vi "Prueba.vi"() -> ()   [LabVIEW 2026]
uses:
  <vilib>/picture/picture.llb/imagedata.ctl
panel:
  out "return code":i32
  out "match + rest of string":string
  out "new picture":picture
  out "standard output":string
  in  "UPLOAD":bool
  in  "DOWNLOAD":bool
  in  "VER IMAGEN":bool
  in  "LEER ARCHIVO":bool
  in  "Single Selection Listbox":i32(listbox)
  out "Lista de archivos":string[](array[string])
  out "Enum":enum16{"ESPERAR", "LIST"}(ring)
  in  "stop":bool
  in  "LISTAR":bool
  in  "IP":string
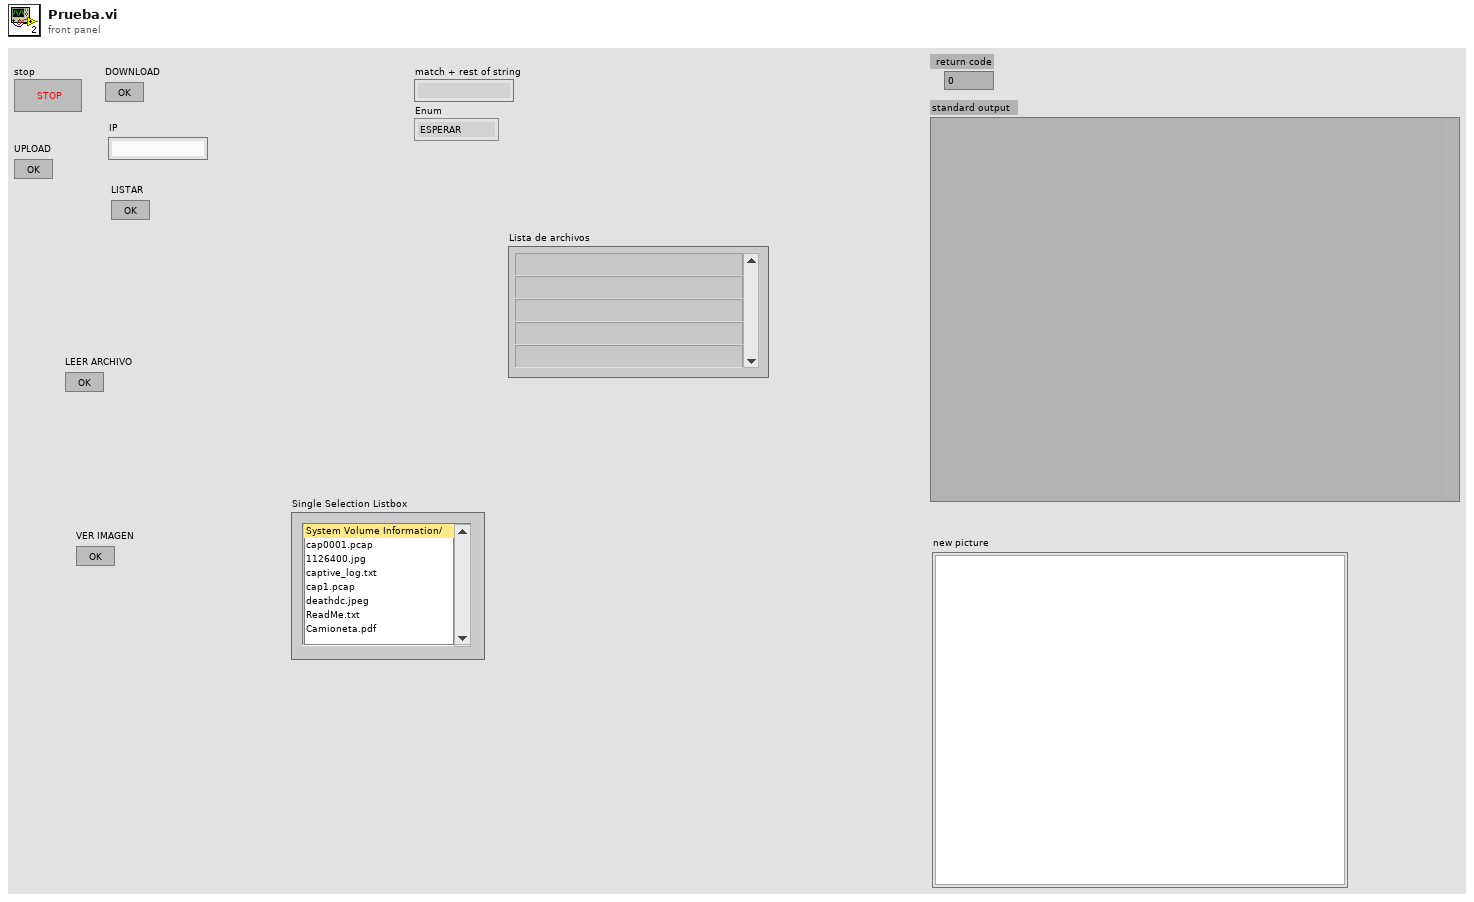
[diagram p1: front panel]
types:
  T1 = enum16{"ESPERAR", "LIST", "ENTRAR", "SUBIR", "DESCARGAR", "UPLOAD"}
  T2 = typedef "imagedata.ctl" = cluster{"image type":i32, "image depth":i32, "image":u8[], "mask":u8[], "colors":u32[], "Rectangle":cluster{"left":i16, "top":i16, "right":i16, "bottom":i16}}
  T3 = typedef "LVBoundsTypeDef.ctl" = cluster{"Width":u32, "Height":u32}
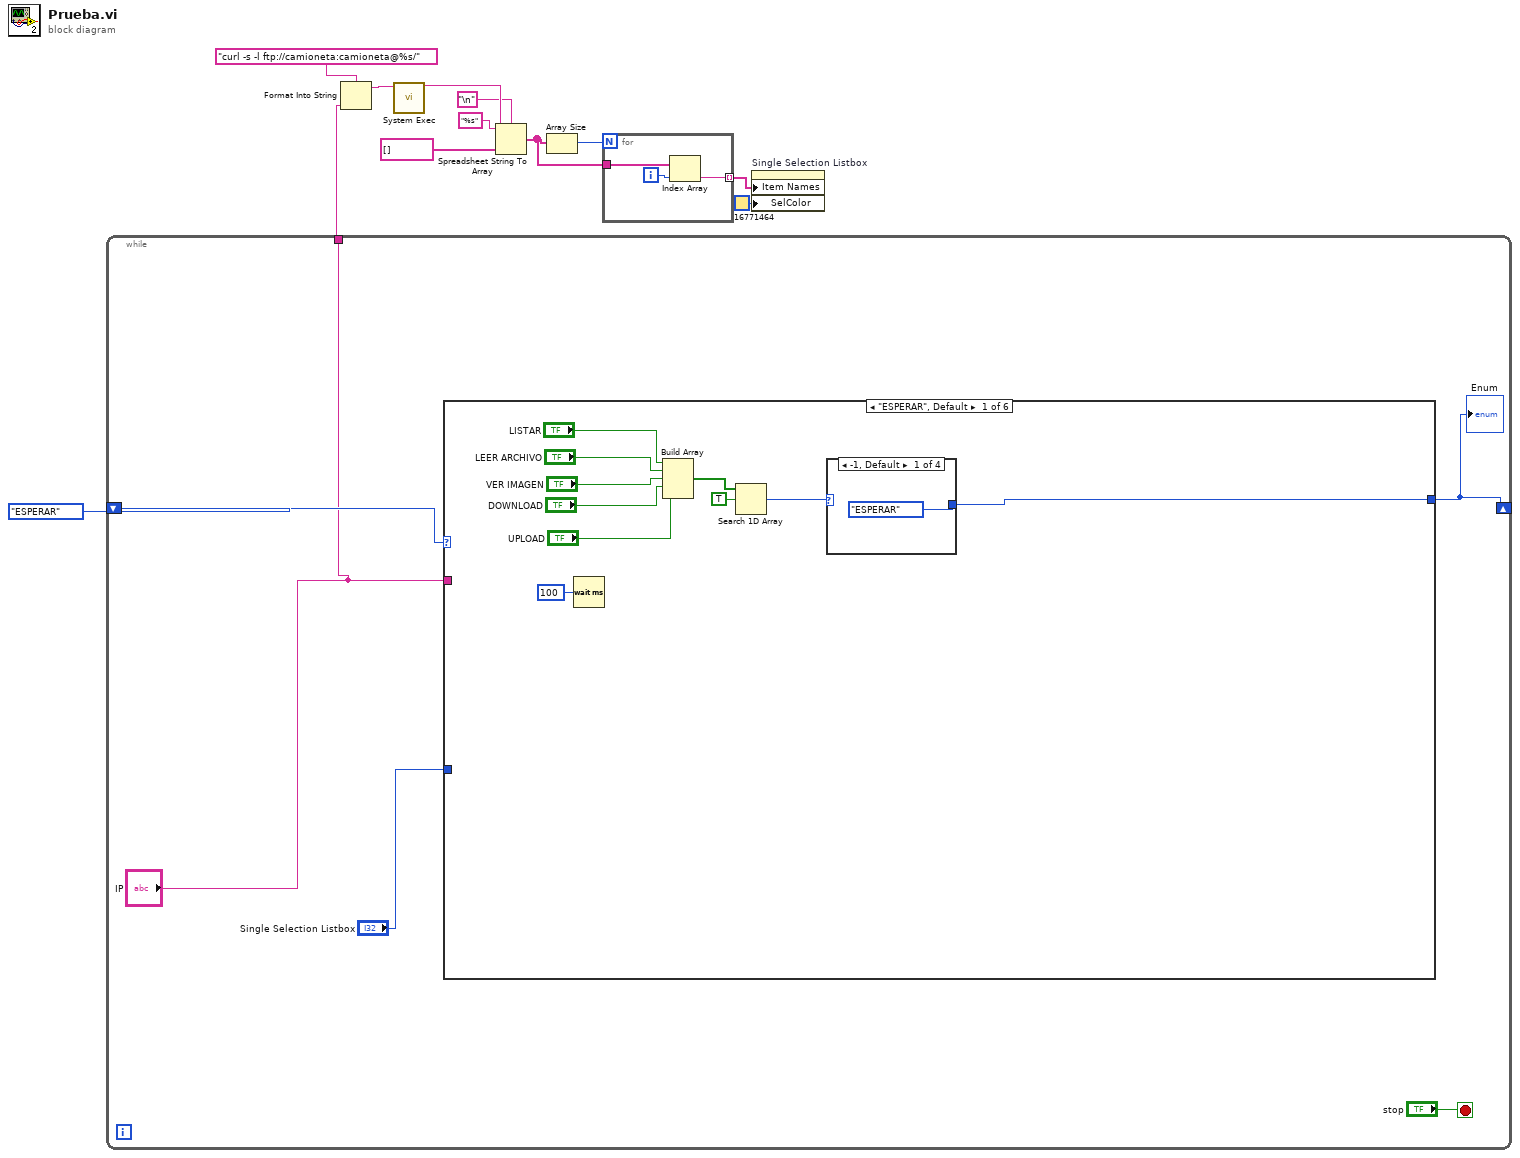
[diagram p0: block diagram]
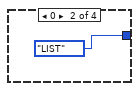
[diagram p2: hidden frame]
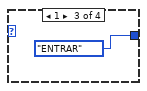
[diagram p3: hidden frame]
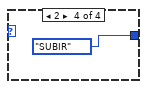
[diagram p4: hidden frame]
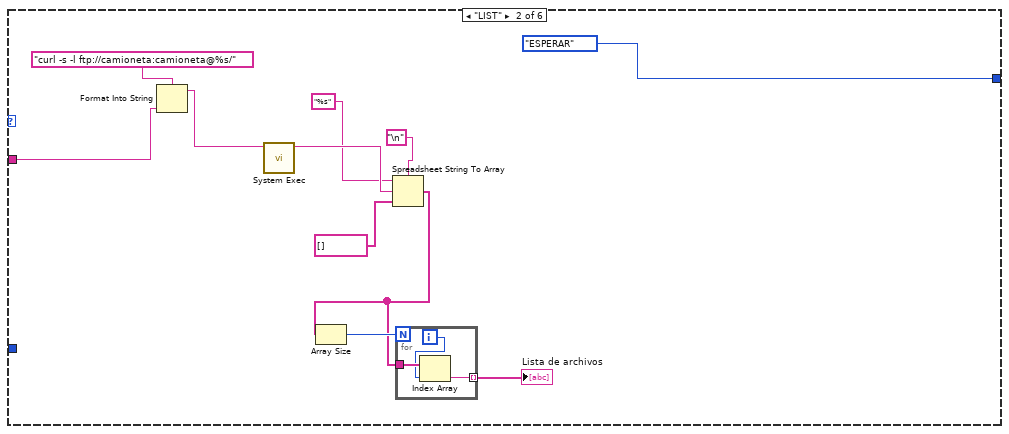
[diagram p5: hidden frame]
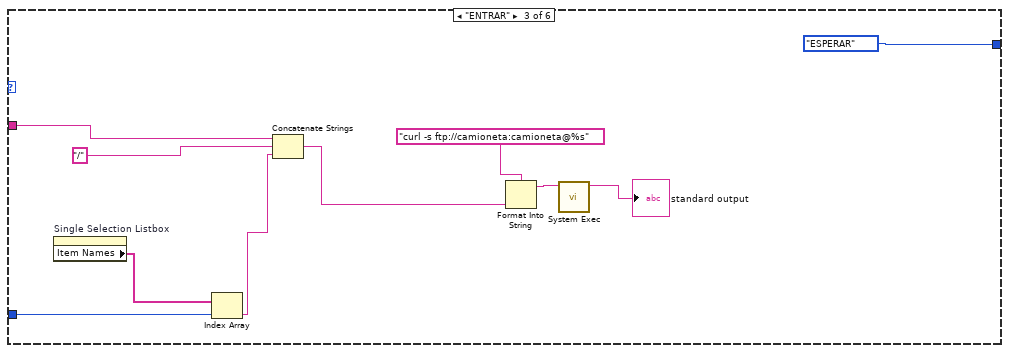
[diagram p6: hidden frame]
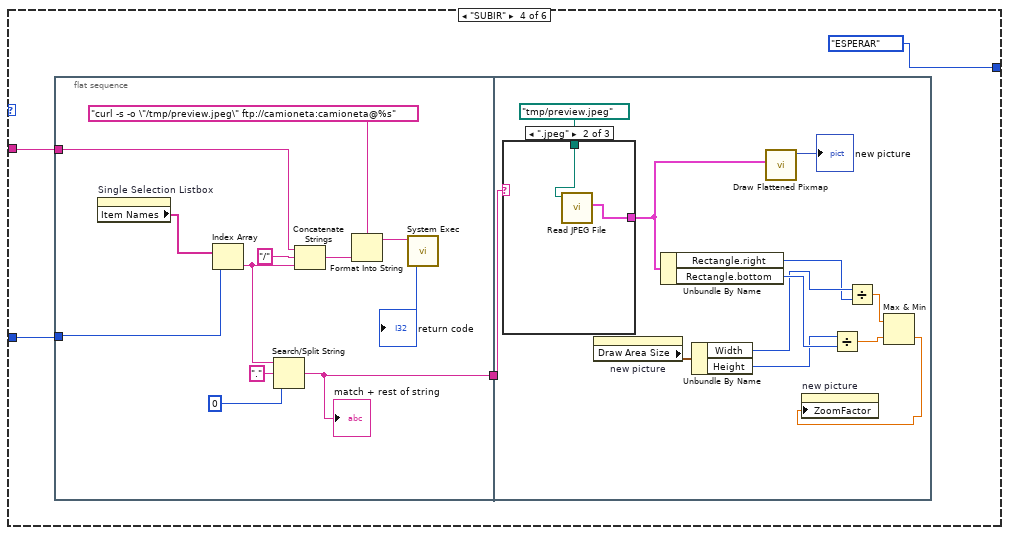
[diagram p7: hidden frame]
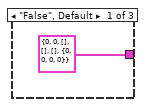
[diagram p8: hidden frame]
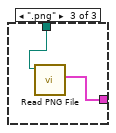
[diagram p9: hidden frame]
diagram:
  n1 = while {
    shift-right: [w16] -> _
    shift-left: T1."ESPERAR" -> [w15]
    tunnel: ["IP"] -> w3
    stop <- "stop" stop-if-true
    n2 = case shown="\"ESPERAR\", Default" w15 {
      tunnel: [w18 T1."ESPERAR" T1."ESPERAR" T1."ESPERAR" _ _] -> w16
      tunnel: "IP" -> [_ w33 w51 w58 _ _]
      tunnel: "Single Selection Listbox" -> [_ _ w46 w59 _ _]
      frame "ESPERAR", Default {
        n3 = Wait (ms)(milliseconds to wait=u32 100) -> ()  [unwired: 1 out]
        n4 = Build Array("LISTAR", "LEER ARCHIVO", "VER IMAGEN", "DOWNLOAD", "UPLOAD") -> (w22:bool[])
        n5 = Search 1D Array(1D array=w22, element=TRUE) -> (index of element=w19:i32)  [unwired: 1 in]
        n6 = case shown="-1, Default" w19 {
          tunnel: [T1."ESPERAR" T1."LIST" T1."ENTRAR" T1."SUBIR"] -> w18
          frame -1, Default {
          }
          frame 0 {
          }
          frame 1 {
          }
          frame 2 {
          }
        }
      }
      frame "LIST" {
        n7 = Format Into String(format string="curl -s -l ftp://camioneta:camioneta@%s/", w33) -> (resulting string=w42:string)  [unwired: 2 in, 1 out]
        n8 = call <vilib>:"System Exec.vi"("command line"=w42) -> ("standard output"=w41:string)  [unwired: 7 in, 3 out]
        n9 = Spreadsheet String To Array(delimiter (Tab)="\n", format string="%s", spreadsheet string=w41, array type (2D Dbl)=string[] []) -> (array=w39:string[])
        n10 = Array Size(array=w39) -> (size(s)=w40:i32)
        n11 = for {
          N: w40 -> [_]
          tunnel: w39 -> [w45]
          tunnel: [w44] -> w32 mode=indexing
          i -> [w43]
          n12 = Index Array(array=w45, index=w43) -> (element=w44:string)
        }
        "Lista de archivos" <- w32
      }
      frame "ENTRAR" {
        n13 = property on="Single Selection Listbox" class="LstBox (strict)"() -> ("Item Names"=w53:string[])  [unwired: 2 in, 2 out]
        n14 = Index Array(array=w53, index=w46) -> (element=w52:string)
        n15 = Concatenate Strings(w51, "/" ("string"), w52) -> (w48:string)
        n16 = Format Into String(format string="curl -s ftp://camioneta:camioneta@%s", w48) -> (resulting string=w49:string)  [unwired: 2 in, 1 out]
        n17 = call <vilib>:"System Exec.vi"("command line"=w49) -> ("standard output"=→"standard output":string)  [unwired: 7 in, 3 out]
      }
      frame "SUBIR" {
        n18 = flat-sequence {
          tunnel: w59 -> [w66]
          tunnel: w58 -> [w65]
          tunnel: [w61] -> w56
          tunnel: w56 -> [w73]
          frame #0 {
            n19 = property on="Single Selection Listbox" class="LstBox (strict)"() -> ("Item Names"=w71:string[])  [unwired: 2 in, 2 out]
            n20 = Index Array(array=w71, index=w66) -> (element=w64:string)
            n21 = Search/Split String(string=w64, search string/char (-)=".", offset (0)=0) -> (match + rest of string=w61:string)  [unwired: 2 out]
            "match + rest of string" <- w61
            n22 = Concatenate Strings(w65, "/" ("string"), w64) -> (w69:string)
            n23 = Format Into String(format string="curl -s -o \"/tmp/preview.jpeg\" ftp://camioneta:camioneta@%s", w69) -> (resulting string=w70:string)  [unwired: 2 in, 1 out]
            n24 = call <vilib>:"System Exec.vi"("command line"=w70) -> ("return code"=→"return code":i32)  [unwired: 7 in, 3 out]
          }
          frame #1 {
            n25 = case shown="\".jpeg\"" w73 {
              tunnel: [T2 {"image type"=0, "image depth"=0, "image"=[], "mask"=[], "colors"=[], "Rectangle"={"left"=0, "top"=0, "right"=0, "bottom"=0}} ("image data") w86 w87] -> w82
              tunnel: path "/tmp/preview.jpeg" ("path to JPEG file") -> [_ w85 w88]
              frame "False", Default {
              }
              frame ".jpeg" {
                n26 = call <vilib>:"Read JPEG File.vi"("path to JPEG file"=w85) -> ("image data"=w86:T2)  [unwired: 8 in, 2 out]
              }
              frame ".png" {
                n27 = call <vilib>:"Read PNG File.vi"("path to PNG file"=w88) -> ("image data"=w87:T2)  [unwired: 8 in, 2 out]
              }
            }
            n28 = property on="new picture" class="Pict"() -> ("Draw Area Size"=w81:T3)  [unwired: 2 in, 2 out]
            n29 = Unbundle By Name(w82) -> ("Rectangle.right"=w77:i16, "Rectangle.bottom"=w80:i16)
            n30 = Unbundle By Name(w81) -> ("Width"=w78:u32, "Height"=w79:u32)
            n31 = call <vilib>:"Draw Flattened Pixmap.vi"("image data"=w82) -> ("new picture"=→"new picture":picture)  [unwired: 8 in]
            n32 = Divide(x=w79, y=w80) -> (x/y=w75:dbl)
            n33 = Divide(x=w78, y=w77) -> (x/y=w76:dbl)
            n34 = Max & Min(x=w76, y=w75) -> (min(x,y)=w74:dbl)  [unwired: 1 out]
            n35 = property on="new picture" class="Pict"("ZoomFactor"=w74) -> ()  [unwired: 2 in, 2 out]
          }
        }
      }
      frame "DESCARGAR" {
      }
      frame "UPLOAD" {
      }
    }
    "Enum" <- w16
  }
  n36 = Format Into String(format string="curl -s -l ftp://camioneta:camioneta@%s/", w3) -> (resulting string=w11:string)  [unwired: 2 in, 1 out]
  n37 = call <vilib>:"System Exec.vi"("command line"=w11) -> ("standard output"=w10:string)  [unwired: 7 in, 3 out]
  n38 = Spreadsheet String To Array(delimiter (Tab)="\n", format string="%s", spreadsheet string=w10, array type (2D Dbl)=string[] []) -> (array=w8:string[])
  n39 = Array Size(array=w8) -> (size(s)=w9:i32)
  n40 = for {
    N: w9 -> [_]
    tunnel: w8 -> [w91]
    tunnel: [w90] -> w2 mode=indexing
    i -> [w89]
    n41 = Index Array(array=w91, index=w89) -> (element=w90:string)
  }
  n42 = property on="Single Selection Listbox" class="LstBox (strict)"("Item Names"=w2, "SelColor"=u32 16771464 ("Selection Color")) -> ()  [unwired: 2 in, 2 out]
